vi "Set All Laser Powers.vi"(8 "error in (no error)":errorcluster, 9 "Power":dbl, 10 "Line Select":bool[](array[boolean]), 11 "Laser Quantum in":refnum<class "Laser.lvclass">) -> (0 "error out":errorcluster, 3 "Laser Quantum out":refnum<class "Laser.lvclass">)   [LabVIEW 2018, in "Laser.lvlib" / "Laser.lvclass"]
uses:
  Laser.lvclass
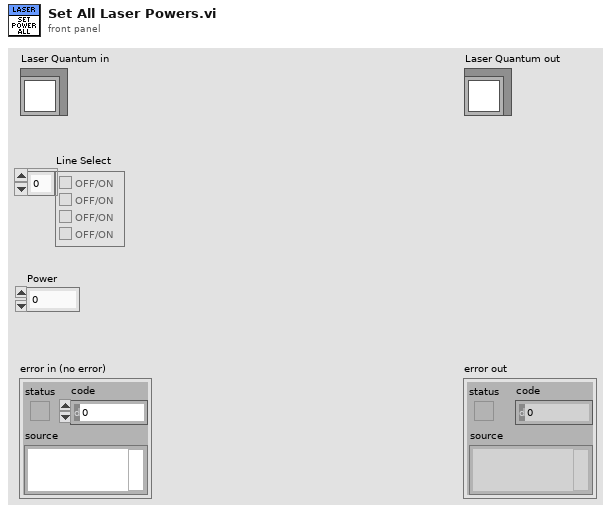
[diagram p1: front panel]
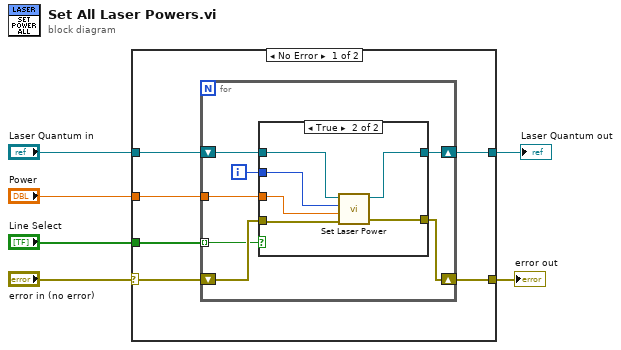
[diagram p0: block diagram]
diagram:
  n1 = case shown="No Error" "error in (no error)" {
    selector: "error in (no error)" -> [w12 w29]
    tunnel: [w11 w29] -> w5
    tunnel: [w7 w28] -> w3
    tunnel: "Laser Quantum in" -> [w8 w28]
    tunnel: "Line Select" -> [w10 _]
    tunnel: "Power" -> [w9 _]
    frame No Error {
      n2 = for {
        shift-right: [w18] -> w11
        shift-left: w12 -> [w19]
        tunnel: w10 -> [w17] mode=indexing
        tunnel: w9 -> [w15]
        shift-right: [w13] -> w7
        shift-left: w8 -> [w14]
        i -> [w16]
        n3 = case shown="True" w17 {
          tunnel: w19 -> [w21 w26]
          tunnel: [w21 w27] -> w18
          tunnel: w16 -> [_ w25]
          tunnel: w15 -> [_ w24]
          tunnel: w14 -> [w20 w23]
          tunnel: [w20 w22] -> w13
          frame False {
          }
          frame True {
            n4 = call-dynamic "Set Laser Power.vi"("error in (no error)"=w26, "Power"=w24, "laser index"=w25, "Laser Quantum in"=w23) -> ("error out"=w27:errorcluster, "Laser Quantum out"=w22:refnum<class "Laser.lvclass">)  [unwired: 6 in]
          }
        }
      }
    }
    frame Error {
    }
  }
  "error out" <- w5
  "Laser Quantum out" <- w3
